vi "enableMonitors.vi"(8 "error in (no error)":errorcluster, 11 "Subnet in":refnum<class "Subnet.lvclass">) -> (0 "error out":errorcluster, 3 "Subnet out":refnum<class "Subnet.lvclass">)   [LabVIEW 2016, in "Subnet.lvclass"]
uses:
  Subnet.lvclass
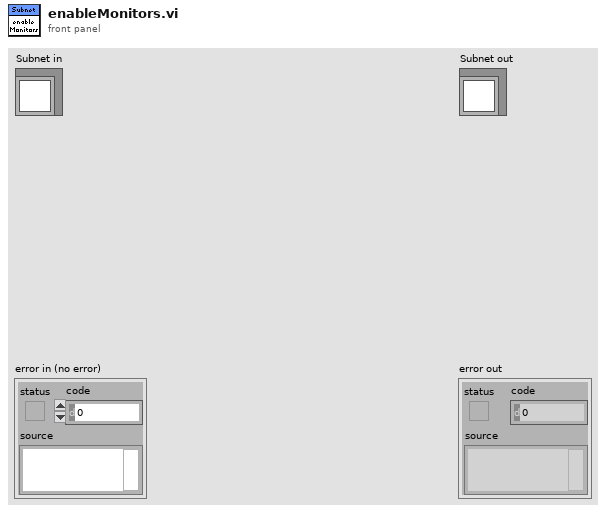
[diagram p1: front panel]
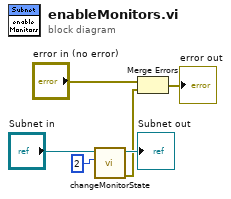
[diagram p0: block diagram]
diagram:
  n1 = call "changeMonitorState.vi"("State"=u16 2, "Subnet in"="Subnet in") -> ("error out"=w1:errorcluster, "Subnet out"=→"Subnet out":refnum<class "Subnet.lvclass">)  [unwired: 8 in]
  n2 = Merge Errors("error in (no error)", w1) -> (→"error out":errorcluster)
